vi "DAQMX send waveform.vi"() -> ()   [LabVIEW 2010]
uses:
  <vilib>/Utility/error.llb/DialogType.ctl
  <vilib>/DAQmx/write.llb/DAQmx Write (Analog Wfm 1Chan NSamp).vi
  <vilib>/DAQmx/create/channels.llb/DAQmx Create Channel (AO-Voltage-Basic).vi
  <vilib>/daqmx/miscellaneous.llb/DAQmx Fill In Error Info.vi
  <vilib>/measure/NI_MABase.lvlib
panel:
  in  "phase 1":dbl=-90.0 format="%.2p"
  in  "?":T1(ring)=enum."Triangle Wave"
  in  "sampling info 1":cluster{"Fs":dbl, "#s":dbl}={"Fs"=1000000.0, "#s"=2500.0} {"Fs" format="%.2p"}
  in  "amplitude 1":dbl=1.0 format="%0.2p"
  in  "frequency 1":dbl=100.0 format="%0.2p"
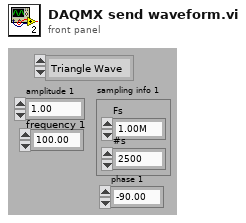
[diagram p1: front panel]
types:
  T1 = enum16{"Sine Wave", "Triangle Wave", "Square Wave", "Sawtooth Wave"}
  T2 = typedef "DialogType.ctl" = u16
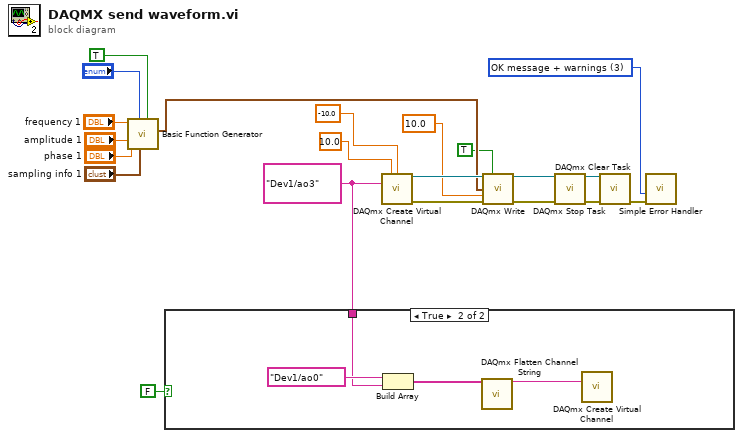
[diagram p0: block diagram]
diagram:
  w10 = tag "Dev1/ao3" ("Physical Channel")
  w16 = T2 3 items=["no dialog", "OK message", "continue or stop message", "OK message + warnings", "continue/stop + warnings"] ("type of dialog (OK msg:1)")
  n1 = call <vilib>:"Basic Function Generator.vi"("reset signal"=TRUE, "sampling info"="sampling info 1", "signal type"="?", "phase"="phase 1", "amplitude"="amplitude 1", "frequency"="frequency 1") -> ("signal out"=w2:waveform(dbl))  [unwired: 3 in, 2 out]
  n2 = case shown="True" FALSE {
    tunnel: w10 -> [_ w24]
    frame False {
    }
    frame True {
      n3 = Build Array(tag "Dev1/ao0" ("physical channels"), w24) -> (w23:tag[])
      n4 = call <vilib>:"DAQmx Flatten Channel String.vi"("names in"=w23) -> ("names out"=w22:string)  [unwired: 13 in, 1 out]
      n5 = call-poly <vilib>:"DAQmx Create Virtual Channel.vi"("physical channels"=w22) -> ()  [unwired: 8 in, 7 out]
    }
  }
  n6 = call-poly <vilib>:"DAQmx Create Virtual Channel.vi"("maximum value"=10.0 ("Maximum Value"), "minimum value"=-10.0 ("Minimum Value"), "physical channels"=w10) -> ("task out"=w18:refnum<k21>, "error out"=w19:errorcluster)  [unwired: 6 in, 5 out]
  n7 = call-poly <vilib>:"DAQmx Write.vi"("task/channels in"=w18, "auto start"=TRUE, "data"=w2, "timeout"=10.0, "error in"=w19) -> ("task out"=w14:refnum<k21>, "error out"=w12:errorcluster)  [unwired: 9 out]
  n8 = call <vilib>:"DAQmx Stop Task.vi"("task/channels in"=w14, "error in"=w12) -> ("task out"=w13:refnum<k21>, "error out"=w11:errorcluster)  [unwired: 12 in]
  n9 = call <vilib>:"DAQmx Clear Task.vi"("task in"=w13, "error in"=w11) -> ("error out"=w15:errorcluster)  [unwired: 13 out]
  n10 = call <vilib>:"Simple Error Handler.vi"("type of dialog (OK msg:1)"=w16, "error in (no error)"=w15) -> ()  [unwired: 8 out]
